vi "Peer Review Tool.vi"() -> ()   [LabVIEW 2020, in "Peer Review.lvclass"]
uses:
  Peer Review.lvclass
  Peer Review.lvclass/Peer Review.ctl
panel:
  in  "Cancel":bool
  out "Automatically Analyze Files?":bool
  out "Progress":dbl(slide) scale=0.0..100.0 scale format="%#.6f"
  out "Status":string
  in  "Run VI Analyzer":bool
  in  "Target":u16(ring)
  in  "Pull Remote Master":bool
  out "Branch Name":string
  in  "Results Directory":path
  in  "Tabs":T1(tab)=enum."File List"
  out "Commit History":string[][](table)
  in  "Files List":i32(listbox)=-1
  out "Git Log":string
  out "Description":string
  in  "Picture":picture
  in  "Review Branch":bool
  in  "Baseline Directory":path
  # "NDAS Peer Review Tool"
  # "Copyright © 2025 United States Government as represented by the Administrator of the National Aeronautics and Space Administration.   All Rights Reserved."
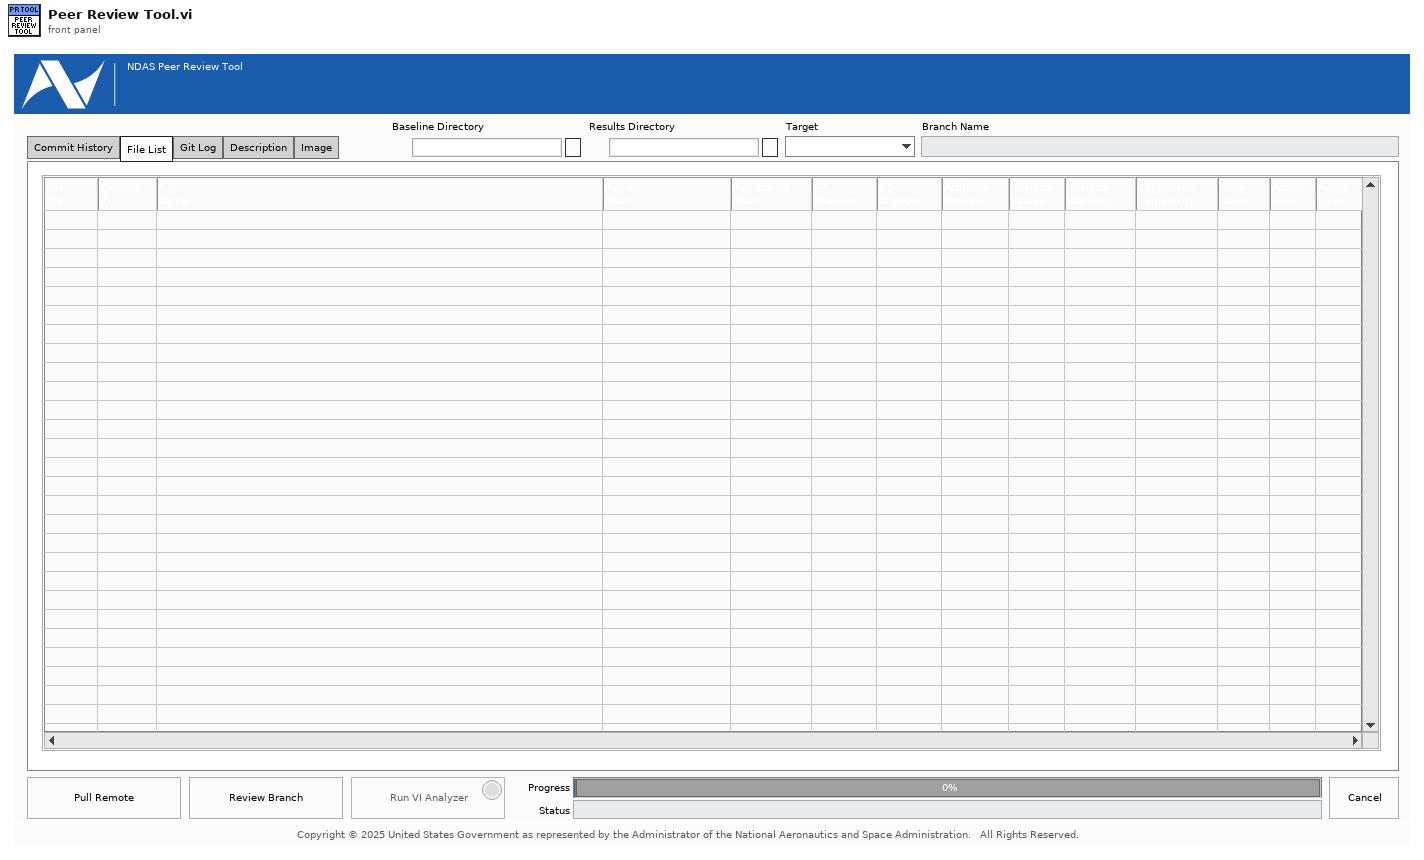
[diagram p1: front panel]
types:
  T1 = enum32{"Commit History", "File List", "Git Log", "Description", "Image"}
  T2 = typedef "LVPoint32TypeDef.ctl" = cluster{"Horizontal":i32, "Vertical":i32}
  T3 = typedef "LVRowAndColumnTypeDef.ctl" = cluster{"Row":i32, "Column":i32}
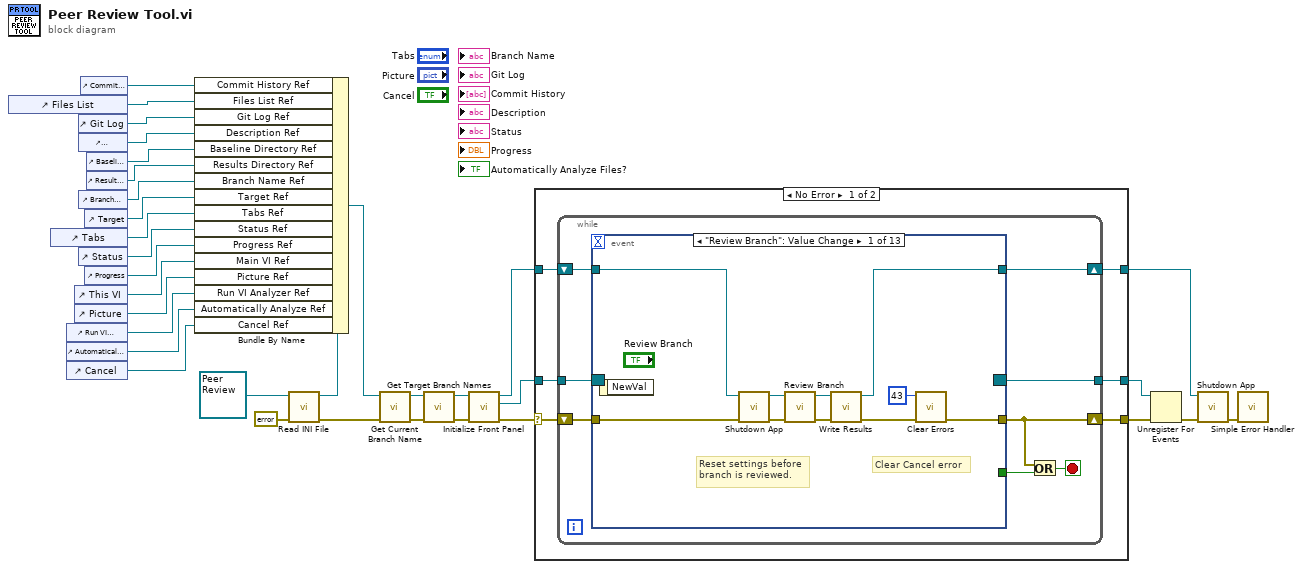
[diagram p0: block diagram]
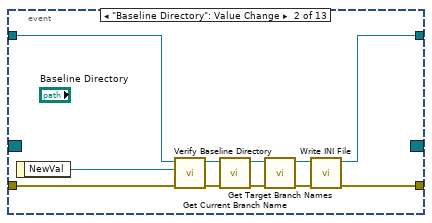
[diagram p2: hidden frame]
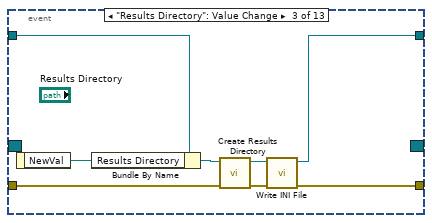
[diagram p3: hidden frame]
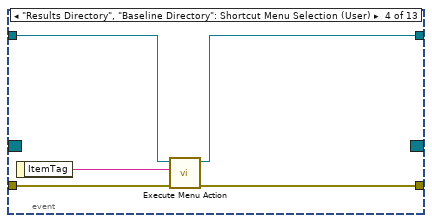
[diagram p4: hidden frame]
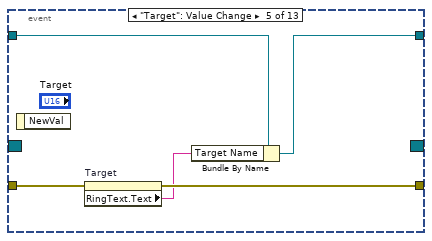
[diagram p5: hidden frame]
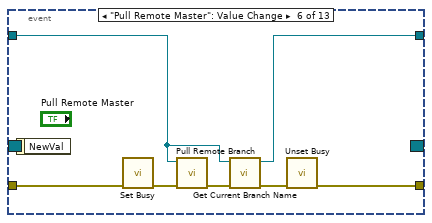
[diagram p6: hidden frame]
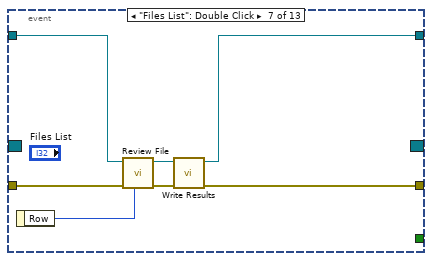
[diagram p7: hidden frame]
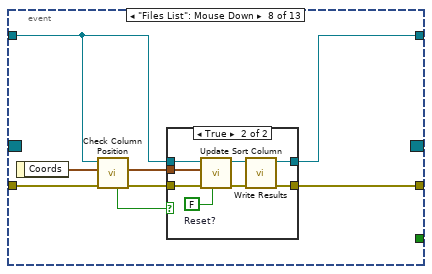
[diagram p8: hidden frame]
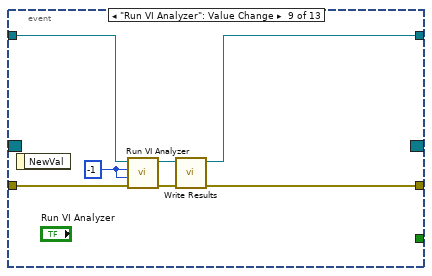
[diagram p10: hidden frame]
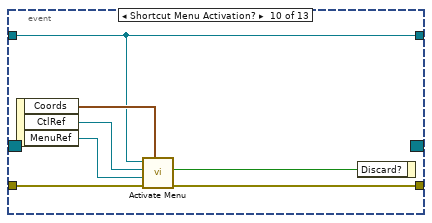
[diagram p11: hidden frame]
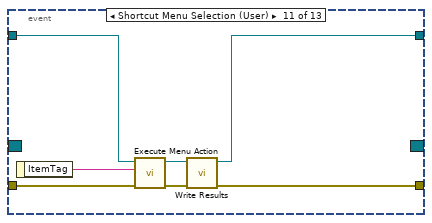
[diagram p12: hidden frame]
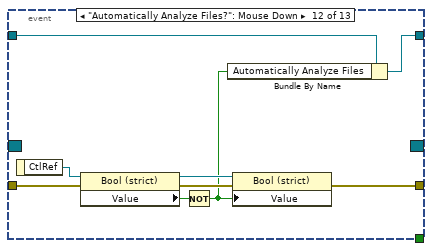
[diagram p13: hidden frame]
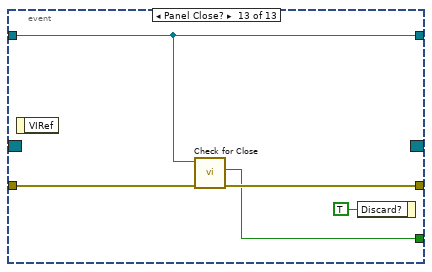
[diagram p14: hidden frame]
diagram:
  n1 = control-ref of="Files List"() -> (w33:refnum<vi>)
  n2 = control-ref of="Tabs"() -> (w13:refnum<vi>)
  n3 = control-ref of="Run VI Analyzer"() -> (w7:refnum<vi>)
  n4 = control-ref of="Automatically Analyze Files?"() -> (w6:refnum<vi>)
  n5 = control-ref of="Cancel"() -> (w1:refnum<vi>)
  n6 = control-ref of="This VI"() -> (w14:refnum<vi>)
  n7 = control-ref of="Picture"() -> (w12:refnum<vi>)
  n8 = control-ref of="Git Log"() -> (w32:refnum<vi>)
  n9 = control-ref of="Description"() -> (w17:refnum<vi>)
  n10 = control-ref of="Branch Name"() -> (w25:refnum<vi>)
  n11 = control-ref of="Status"() -> (w16:refnum<vi>)
  n12 = control-ref of="Commit History"() -> (w29:refnum<vi>)
  n13 = control-ref of="Target"() -> (w26:refnum<vi>)
  n14 = control-ref of="Progress"() -> (w15:refnum<vi>)
  n15 = control-ref of="Baseline Directory"() -> (w11:refnum<vi>)
  n16 = control-ref of="Results Directory"() -> (w3:refnum<vi>)
  n17 = call "Read INI File.vi"("error in"=errorcluster {"status"=FALSE, "code"=0, "source"=""} ("error out"), "Peer Review in"=refnum<class "Peer Review.lvclass"> refnum) -> ("error out"=w2:errorcluster, "Peer Review out"=w23:refnum<class "Peer Review.lvclass">)  [unwired: 8 in]
  n18 = Bundle By Name(cluster=w23, "Commit History Ref"=w29, "Files List Ref"=w33, "Git Log Ref"=w32, "Description Ref"=w17, "Baseline Directory Ref"=w11, "Results Directory Ref"=w3, "Branch Name Ref"=w25, "Target Ref"=w26, "Tabs Ref"=w13, "Status Ref"=w16, "Progress Ref"=w15, "Main VI Ref"=w14, "Picture Ref"=w12, "Run VI Analyzer Ref"=w7, "Automatically Analyze Ref"=w6, "Cancel Ref"=w1) -> (w22:refnum<class "Peer Review.lvclass">)
  n19 = call "Get Current Branch Name.vi"("error in"=w2, "Peer Review in"=w22) -> ("error out"=w21:errorcluster, "Peer Review out"=w24:refnum<class "Peer Review.lvclass">)  [unwired: 8 in]
  n20 = call "Get Target Branch Names.vi"("error in"=w21, "Peer Review in"=w24) -> ("error out"=w9:errorcluster, "Peer Review out"=w10:refnum<class "Peer Review.lvclass">)  [unwired: 8 in]
  n21 = call "Initialize Front Panel.vi"("error in"=w9, "Peer Review in"=w10) -> ("error out"=w4:errorcluster, "Event Registration Refnum"=w5:refnum<event-registration>, "Peer Review out"=w8:refnum<class "Peer Review.lvclass">)  [unwired: 7 in]
  n22 = case shown="No Error" w4 {
    selector: w4 -> [w38 w155]
    tunnel: [w39 w156] -> w30
    tunnel: w5 -> [w37 w154]
    tunnel: [w36 w154] -> w20
    tunnel: [w35 w155] -> w19
    tunnel: w8 -> [w34 w156]
    frame No Error {
      n23 = while {
        shift-right: [w46] -> w35
        shift-left: w38 -> [w47]
        shift-right: [w42] -> w39
        shift-left: w34 -> [w43]
        tunnel: w37 -> [w41]
        tunnel: [w40] -> w36
        stop <- w44 stop-if-true
        n24 = event shown="[0] \"Review Branch\": Value Change" {
          selector: w41 -> [_ _ _ _ _ _ _ _ _ _ _ _ _]
          dyn-events: [_ _ _ _ _ _ _ _ _ _ _ _ _] -> w40
          timeout: _ -> [_ _ _ _ _ _ _ _ _ _ _ _ _]
          tunnel: w47 -> [w54 w63 w74 w81 w83 w88 w98 w105 w124 w132 w139 w148 w151]
          tunnel: [w49 w67 w69 w80 w84 w92 w96 w107 w121 w128 w135 w143 w152] -> w46
          tunnel: [_ _ _ _ _ _ _ _ _ _ _ _ w149] -> w45
          tunnel: [w52 w68 w71 w78 w85 w91 w94 w108 w119 w126 w133 w140 w150] -> w42
          tunnel: w43 -> [w55 w66 w76 w79 w86 w87 w100 w104 w125 w126 w138 w142 w150]
          event "Review Branch": Value Change {
            # "Clear Cancel error"
            # "Reset settings before\nbranch is reviewed."
            n25 = event-data() -> ()  [unwired: 1 in, 1 out]
            n26 = call "Shutdown App.vi"("error in"=w54, "Peer Review in"=w55) -> ("error out"=w57:errorcluster, "Peer Review out"=w56:refnum<class "Peer Review.lvclass">)  [unwired: 8 in]
            n27 = call "Review Branch.vi"("error in"=w57, "Peer Review in"=w56) -> ("error out"=w51:errorcluster, "Peer Review out"=w53:refnum<class "Peer Review.lvclass">)  [unwired: 8 in]
            n28 = call "Write Results.vi"("error in"=w51, "Peer Review in"=w53) -> ("error out"=w50:errorcluster, "Peer Review out"=w52:refnum<class "Peer Review.lvclass">)  [unwired: 8 in]
            n29 = call <vilib>:"Clear Errors.vi"("error in (no error)"=w50, "specific error code to clear (0: all)"=43) -> ("error out"=w49:errorcluster)  [unwired: 4 in, 1 out]
          }
          event "Baseline Directory": Value Change {
            n30 = event-data() -> ("NewVal"=w62:path)  [unwired: 1 in]
            n31 = call "Verify Baseline Directory.vi"("error in"=w63, "Baseline Directory"=w62, "Peer Review in"=w66) -> ("error out"=w64:errorcluster, "Peer Review out"=w65:refnum<class "Peer Review.lvclass">)  [unwired: 7 in]
            n32 = call "Get Current Branch Name.vi"("error in"=w64, "Peer Review in"=w65) -> ("error out"=w59:errorcluster, "Peer Review out"=w61:refnum<class "Peer Review.lvclass">)  [unwired: 8 in]
            n33 = call "Get Target Branch Names.vi"("error in"=w59, "Peer Review in"=w61) -> ("error out"=w58:errorcluster, "Peer Review out"=w60:refnum<class "Peer Review.lvclass">)  [unwired: 8 in]
            n34 = call "Write INI File.vi"("error in"=w58, "Peer Review in"=w60) -> ("error out"=w67:errorcluster, "Peer Review out"=w68:refnum<class "Peer Review.lvclass">)  [unwired: 8 in]
          }
          event "Results Directory": Value Change {
            n35 = event-data() -> ("NewVal"=w75:path)  [unwired: 1 in]
            n36 = Bundle By Name(cluster=w76, "Results Directory"=w75) -> (w73:refnum<class "Peer Review.lvclass">)
            n37 = call "Create Results Directory.vi"("error in"=w74, "Peer Review in"=w73) -> ("error out"=w70:errorcluster, "Peer Review out"=w72:refnum<class "Peer Review.lvclass">)  [unwired: 8 in]
            n38 = call "Write INI File.vi"("error in"=w70, "Peer Review in"=w72) -> ("error out"=w69:errorcluster, "Peer Review out"=w71:refnum<class "Peer Review.lvclass">)  [unwired: 8 in]
          }
          event "Results Directory", "Baseline Directory": Shortcut Menu Selection (User) {
            n39 = event-data() -> ("ItemTag"=w77:string)  [unwired: 1 in]
            n40 = call "Execute Menu Action.vi"("error in"=w81, "Item Tag"=w77, "Peer Review in"=w79) -> ("error out"=w80:errorcluster, "Peer Review out"=w78:refnum<class "Peer Review.lvclass">)  [unwired: 7 in]
          }
          event "Target": Value Change {
            n41 = event-data() -> ()  [unwired: 1 in, 1 out]
            n42 = property on="Target" class="Ring (strict)"(error in=w83) -> (error out=w84:errorcluster, "RingText.Text"=w82:string)  [unwired: 1 in, 1 out]
            n43 = Bundle By Name(cluster=w86, "Target Name"=w82) -> (w85:refnum<class "Peer Review.lvclass">)
          }
          event "Pull Remote Master": Value Change {
            n44 = event-data() -> ()  [unwired: 1 in, 1 out]
            n45 = call <vilib>:"Set Busy.vi"("error in (no error)"=w88) -> ("error out"=w93:errorcluster)  [unwired: 9 in, 1 out]
            n46 = call "Pull Remote Branch.vi"("error in"=w93, "Peer Review"=w87) -> ("error out"=w90:errorcluster)  [unwired: 9 in]
            n47 = call "Get Current Branch Name.vi"("error in"=w90, "Peer Review in"=w87) -> ("error out"=w89:errorcluster, "Peer Review out"=w91:refnum<class "Peer Review.lvclass">)  [unwired: 8 in]
            n48 = call <vilib>:"Unset Busy.vi"("error in (no error)"=w89) -> ("error out"=w92:errorcluster)  [unwired: 10 in]
          }
          event "Files List": Double Click {
            n49 = event-data() -> ("Row"=w99:i32)  [unwired: 1 in]
            n50 = call "Review File.vi"("Row Index"=w99, "error in"=w98, "Peer Review in"=w100) -> ("error out"=w97:errorcluster, "Peer Review out"=w95:refnum<class "Peer Review.lvclass">)  [unwired: 7 in]
            n51 = call "Write Results.vi"("error in"=w97, "Peer Review in"=w95) -> ("error out"=w96:errorcluster, "Peer Review out"=w94:refnum<class "Peer Review.lvclass">)  [unwired: 8 in]
          }
          event "Files List": Mouse Down {
            n52 = event-data() -> ("Coords"=w106:T2)  [unwired: 1 in]
            n53 = call "Check Column Position.vi"("error in"=w105, "Coords"=w106, "Peer Review"=w104) -> ("error out"=w102:errorcluster, "Cell Position"=w103:T3, "Valid Position?"=w101:bool)  [unwired: 6 in]
            n54 = case shown="True" w101 {
              tunnel: [w110 w116] -> w108
              tunnel: [w109 w114] -> w107
              tunnel: w104 -> [w110 w113]
              tunnel: w103 -> [_ w112]
              tunnel: w102 -> [w109 w111]
              frame False {
              }
              frame True {
                w118 = FALSE  # Reset?
                n55 = call "Update Sort Column.vi"("Reset?"=w118, "error in"=w111, "Cell Position"=w112, "Peer Review in"=w113) -> ("error out"=w115:errorcluster, "Peer Review out"=w117:refnum<class "Peer Review.lvclass">)  [unwired: 6 in]
                n56 = call "Write Results.vi"("error in"=w115, "Peer Review in"=w117) -> ("error out"=w114:errorcluster, "Peer Review out"=w116:refnum<class "Peer Review.lvclass">)  [unwired: 8 in]
              }
            }
          }
          event "Run VI Analyzer": Value Change {
            w123 = -1 ("Commit ID")
            n57 = event-data() -> ()  [unwired: 1 in, 1 out]
            n58 = call "Run VI Analyzer.vi"("error in"=w124, "File ID"=w123, "Commit ID"=w123, "Peer Review in"=w125) -> ("error out"=w122:errorcluster, "Peer Review out"=w120:refnum<class "Peer Review.lvclass">)  [unwired: 6 in]
            n59 = call "Write Results.vi"("error in"=w122, "Peer Review in"=w120) -> ("error out"=w121:errorcluster, "Peer Review out"=w119:refnum<class "Peer Review.lvclass">)  [unwired: 8 in]
          }
          event Shortcut Menu Activation? {
            n60 = event-data() -> ("Coords"=w129:T2, "CtlRef"=w130:refnum<vi>, "MenuRef"=w131:refnum<k9>)  [unwired: 1 in]
            n61 = call "Activate Menu.vi"("Coords"=w129, "error in"=w132, "Menu Ref"=w131, "Control Ref"=w130, "Peer Review"=w126) -> ("error out"=w128:errorcluster, "Discard?"=w127:bool)  [unwired: 5 in]
            n62 = event-data("Discard?"=w127) -> ()  [unwired: 1 in, 1 out]
          }
          event Shortcut Menu Selection (User) {
            n63 = event-data() -> ("ItemTag"=w137:string)  [unwired: 1 in]
            n64 = call "Execute Menu Action.vi"("error in"=w139, "Item Tag"=w137, "Peer Review in"=w138) -> ("error out"=w136:errorcluster, "Peer Review out"=w134:refnum<class "Peer Review.lvclass">)  [unwired: 7 in]
            n65 = call "Write Results.vi"("error in"=w136, "Peer Review in"=w134) -> ("error out"=w135:errorcluster, "Peer Review out"=w133:refnum<class "Peer Review.lvclass">)  [unwired: 8 in]
          }
          event "Automatically Analyze Files?": Mouse Down {
            n66 = event-data() -> ("CtlRef"=w147:refnum<vi>)  [unwired: 1 in]
            n67 = property class="Bool (strict)"(reference=w147, error in=w148) -> (reference out=w145:refnum<vi>, error out=w146:errorcluster, "Value"=w144:bool)
            n68 = Not(x=w144) -> (.not. x?=w141:bool)
            n69 = Bundle By Name(cluster=w142, "Automatically Analyze Files"=w141) -> (w140:refnum<class "Peer Review.lvclass">)
            n70 = property class="Bool (strict)"(reference=w145, error in=w146, "Value"=w141) -> (error out=w143:errorcluster)  [unwired: 1 out]
          }
          event Panel Close? {
            n71 = event-data() -> ()  [unwired: 1 in, 1 out]
            n72 = call "Check for Close.vi"("error in"=w151, "Peer Review"=w150) -> ("error out"=w152:errorcluster, "Close?"=w149:bool)  [unwired: 8 in]
            n73 = event-data ("Event Filter Node")("Discard?"=TRUE) -> ()  [unwired: 1 in, 1 out]
          }
        }
        n74 = Or(x=w46, y=w45) -> (x .or. y?=w44:bool)
      }
    }
    frame Error {
    }
  }
  n75 = Unregister For Events(event registration refnum=w20, error in=w19) -> (error out=w18:errorcluster)
  n76 = call "Shutdown App.vi"("error in"=w18, "Peer Review in"=w30) -> ("error out"=w31:errorcluster)  [unwired: 8 in, 1 out]
  n77 = call <vilib>:"Simple Error Handler.vi"("error in (no error)"=w31) -> ()  [unwired: 4 in, 5 out]
